vi "Write RangeMax.vi"(8 "error in (no error)":errorcluster, 10 "RangeMax":dbl, 11 "Configure RangeMax Msg in":refnum<class "Configure RangeMax Msg.lvclass">) -> (0 "error out":errorcluster, 3 "Configure RangeMax Msg out":refnum<class "Configure RangeMax Msg.lvclass">)   [LabVIEW 2015, in "CS++Motor.lvlib" / "Configure RangeMax Msg.lvclass"]
uses:
  Configure RangeMax Msg.lvclass
  Configure RangeMax Msg.lvclass/Configure RangeMax Msg.ctl
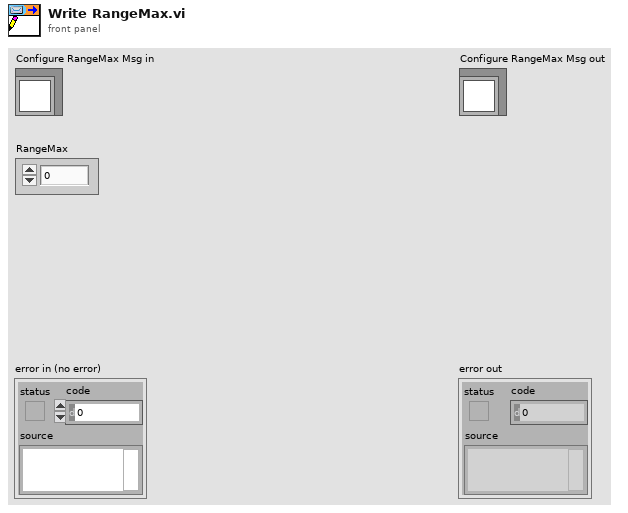
[diagram p1: front panel]
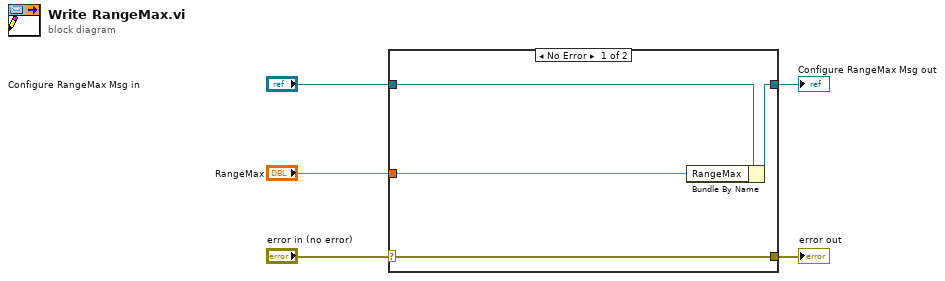
[diagram p0: block diagram]
diagram:
  n1 = case shown="No Error" "error in (no error)" {
    selector: "error in (no error)" -> [w9 w10]
    tunnel: [w9 w10] -> w4
    tunnel: [w7 w11] -> w2
    tunnel: "Configure RangeMax Msg in" -> [w8 w11]
    tunnel: "RangeMax" -> [w6 _]
    frame No Error {
      n2 = Bundle By Name(cluster=w8, "RangeMax"=w6) -> (w7:refnum<class "Configure RangeMax Msg.lvclass">)
    }
    frame Error {
    }
  }
  "error out" <- w4
  "Configure RangeMax Msg out" <- w2
